vi "Array_Shuffle.vi"(4 "Array":sgl[][](array[numeric])) -> (1 "shuffled array":dbl[][](array[numeric]))   [LabVIEW 2020]
uses:
  0e925cb2-5899-4e16-8ee9-684c9ed387e0.vi
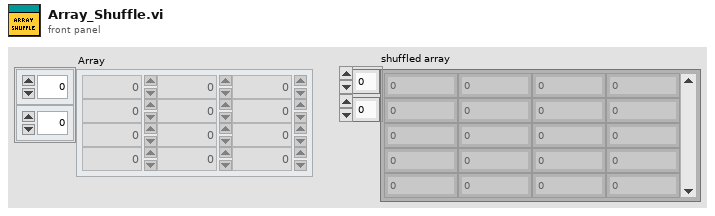
[diagram p1: front panel]
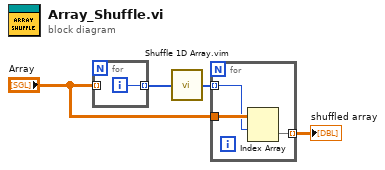
[diagram p0: block diagram]
diagram:
  n1 = for {
    tunnel: "Array" -> [_] mode=indexing
    tunnel: [w5] -> w2 mode=indexing
    i -> [w5]
  }
  n2 = call "Shuffle 1D Array.vim"("array"=w2) -> ("shuffled array"=w1:i32[])  [unwired: 4 in]
  n3 = for {
    tunnel: w1 -> [w7] mode=indexing
    tunnel: "Array" -> [w8]
    tunnel: [w6] -> w4 mode=indexing
    n4 = Index Array(array=w8, index (row)=w7) -> (element=w6:sgl[])  [unwired: 1 in]
  }
  "shuffled array" <- w4
